vi "Model.vi"(8 "error in (no error)":errorcluster, 11 "Sensor in":refnum<class "Sensor.lvclass">) -> (0 "error out":errorcluster, 2 "Model":string, 3 "Sensor out":refnum<class "Sensor.lvclass">)   [LabVIEW 2020, in "VolatusConfig.lvlib" / "Sensor.lvclass"]
uses:
  Sensor.lvclass
  C:/dev/lv20CE/relink/lv-volatus/VolatusConfig/VolatusConfigElement/VolatusConfigElement.lvclass
  VolatusConfigElement/VolatusConfigElement.lvclass/VolatusConfigElement.ctl
  VolatusConfigElement/Element.vi
  VolatusConfigElement/VolatusConfigElement.lvclass
  lv-cdm/CDM-Config/Config Element/Config Element.lvclass
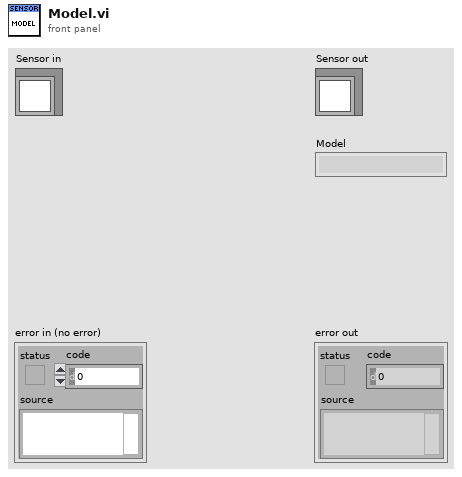
[diagram p1: front panel]
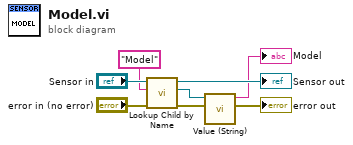
[diagram p0: block diagram]
diagram:
  n1 = call "Lookup Child by Name.vi"("error in (no error)"="error in (no error)", "Child Name"="Model", "VolatusConfigElement in"="Sensor in") -> ("error out"=w4:errorcluster, "Child"=w3:refnum<class "Config Element.lvclass">, "VolatusConfigElement out"=→"Sensor out":refnum<class "Sensor.lvclass">)  [unwired: 5 in, 1 out]
  n2 = call "Value (String).vi"("error in (no error)"=w4, "Config Element in"=w3) -> ("error out"=→"error out":errorcluster, "String Value"=→"Model":string)  [unwired: 8 in]
